vi "ArmGetUpDown.vi"() -> (2 "ArmUpDown":bool)   [LabVIEW 2020]
doc: "Arm Up Down Getter\nOutputs:\n--ArmUpDown--Boolean--"
uses:
  ArmGlobal.vi
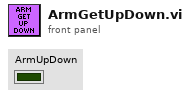
[diagram p1: front panel]
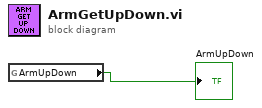
[diagram p0: block diagram]
diagram:
  n1 = global read "ArmGlobal.vi" "ArmUpDown"() -> (→"ArmUpDown":bool)
